vi "Queue Insert.vi"(6 "timeout(ms: -1)":i32=-1, 7 "at front (F)":bool caption="at front? (F)", 8 "error in (no error)":errorcluster, 9 "data":variant, 10 "event":string, 11 "queue name":string) -> (0 "error out":errorcluster, 3 "timeout？":bool)   [LabVIEW 2020]
uses:
  Control/Queue Data.ctl
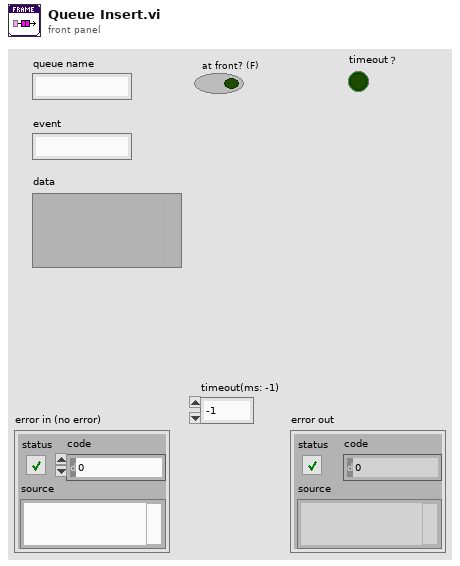
[diagram p1: front panel]
types:
  T1 = typedef "Queue Data.ctl" = cluster{"event":string, "data":variant}
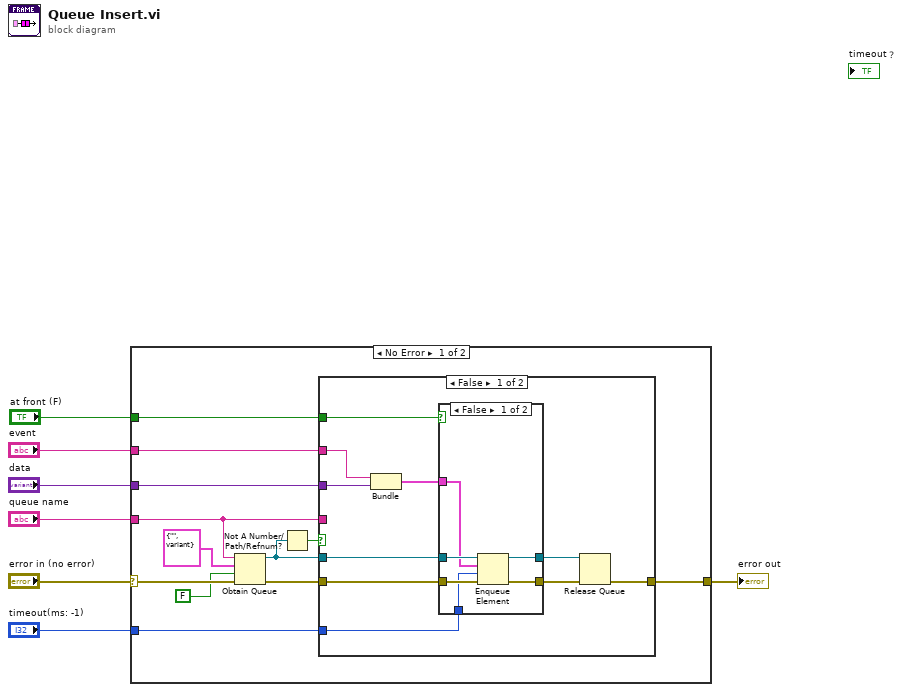
[diagram p0: block diagram]
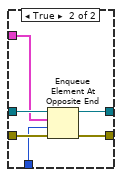
[diagram p2: hidden frame]
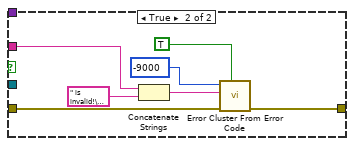
[diagram p3: hidden frame]
diagram:
  n1 = case shown="No Error" "error in (no error)" {
    selector: "error in (no error)" -> [w19 w49]
    tunnel: [w13 w49] -> w6
    tunnel: "queue name" -> [w14 _]
    tunnel: "at front (F)" -> [w12 _]
    tunnel: "event" -> [w9 _]
    tunnel: "data" -> [w8 _]
    tunnel: "timeout(ms: -1)" -> [w10 _]
    frame No Error {
      n2 = Obtain Queue(name (unnamed)=w14, element data type=T1 {"event"="", "data"=variant} ("Cluster"), create if not found? (T)=FALSE, error in (no error)=w19) -> (queue out=w11:refnum<queue>, error out=w16:errorcluster)  [unwired: 1 in, 1 out]
      n3 = Not A Number/Path/Refnum?(number/path/refnum=w11) -> (NaN/Path/Refnum?=w15:bool)
      n4 = case shown="False" w15 {
        tunnel: w16 -> [w27 w44]
        tunnel: w14 -> [_ w43]
        tunnel: [w21 w42] -> w13
        tunnel: w12 -> [w29 _]
        tunnel: w11 -> [w28 _]
        tunnel: w10 -> [w26 _]
        tunnel: w9 -> [w24 _]
        tunnel: w8 -> [w25 _]
        frame False {
          n5 = Bundle("event"=w24, "data"=w25) -> (w23:cluster{"event":string, "data":variant})  [unwired: 1 in]
          n6 = case shown="False" w29 {
            tunnel: [w34 w41] -> w22
            tunnel: w28 -> [w33 w40]
            tunnel: w27 -> [w35 w39]
            tunnel: w26 -> [w32 w37]
            tunnel: w23 -> [w31 w38]
            tunnel: [w30 w36] -> w20
            frame False {
              n7 = Enqueue Element(queue=w33, element=w31, timeout in ms (-1)=w32, error in (no error)=w35) -> (queue out=w30:refnum<queue>, error out=w34:errorcluster)  [unwired: 1 out]
            }
            frame True {
              n8 = Enqueue Element At Opposite End(queue=w40, element=w38, timeout in ms (-1)=w37, error in (no error)=w39) -> (queue out=w36:refnum<queue>, error out=w41:errorcluster)  [unwired: 1 out]
            }
          }
          n9 = Release Queue(queue=w20, error in (no error)=w22) -> (error out=w21:errorcluster)  [unwired: 1 in, 2 out]
        }
        frame True {
          n10 = Concatenate Strings(w43, " is invalid!\nEnsure the queue has been created!" ("字符串")) -> (w46:string)
          n11 = call <vilib>:"Error Cluster From Error Code.vi"("show call chain? (False)"=TRUE, "error in (no error)"=w44, "error message (\"\")"=w46, "error code (0)"=-9000) -> ("error out"=w42:errorcluster)  [unwired: 5 in]
        }
      }
    }
    frame Error {
    }
  }
  "error out" <- w6
